vi "Read Measurements.vi"(8 "error in (no error)":errorcluster, 11 "SPECAN_IQSLOT in":refnum<class "SPECAN_IQSLOT.lvclass">) -> (0 "error out":errorcluster, 2 "Measurements":string, 3 "SPECAN_IQSLOT out":refnum<class "SPECAN_IQSLOT.lvclass">)   [LabVIEW 2018, in "SPECAN_IQSLOT.lvlib" / "SPECAN_IQSLOT.lvclass"]
uses:
  SPECAN_IQSLOT.lvclass
  SPECAN_IQSLOT.lvclass/SPECAN_IQSLOT.ctl
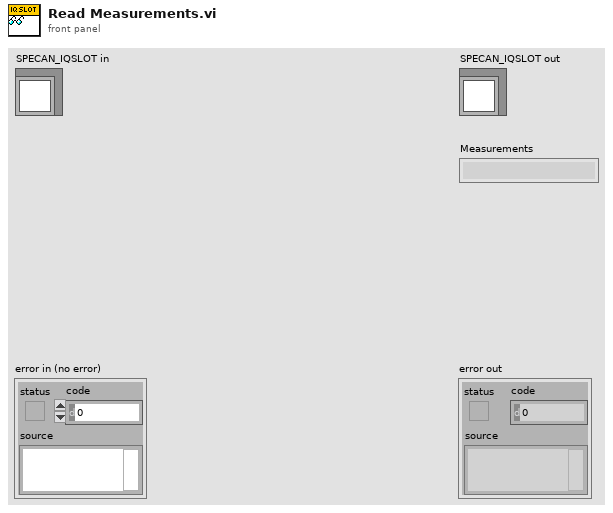
[diagram p1: front panel]
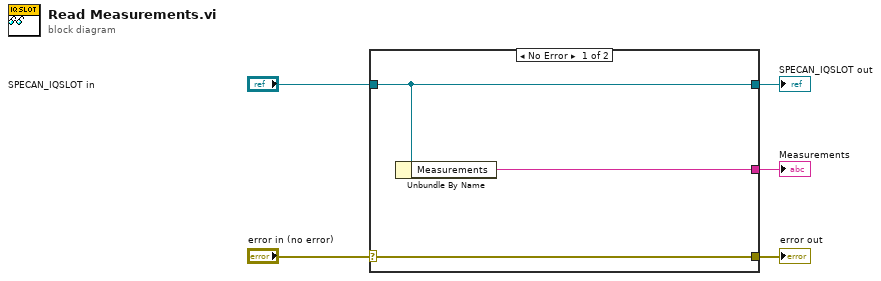
[diagram p0: block diagram]
diagram:
  n1 = case shown="No Error" "error in (no error)" {
    selector: "error in (no error)" -> [w8 w9]
    tunnel: [w8 w9] -> w4
    tunnel: [w7 w10] -> w2
    tunnel: "SPECAN_IQSLOT in" -> [w7 w10]
    tunnel: [w6 _] -> w1
    frame No Error {
      n2 = Unbundle By Name(w7) -> ("Measurements"=w6:string)
    }
    frame Error {
    }
  }
  "error out" <- w4
  "SPECAN_IQSLOT out" <- w2
  "Measurements" <- w1
